vi "arm_delta.vi"(8 "Compliance [V]":dbl=0.5 format="%#_6f", 9 "DELAY [sec]":dbl=0.002 format="%#_6e", 10 "I-HIGH [A]":dbl=0.0001 format="%#_6e", 11 "Keithley":refnum<visa-resource-name>="GPIB1::20::INSTR") -> (3 "number":i32)   [LabVIEW 2019]
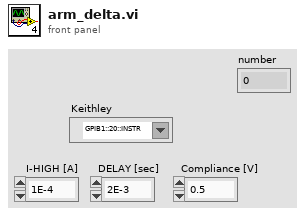
[diagram p1: front panel]
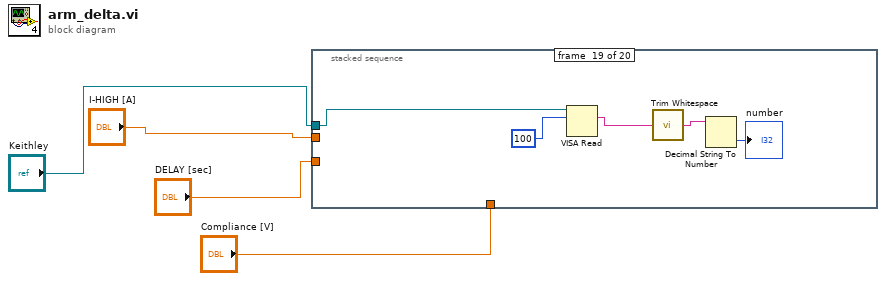
[diagram p0: block diagram]
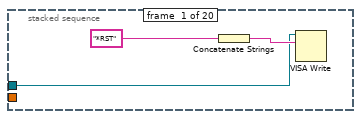
[diagram p2: hidden frame]
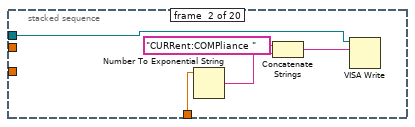
[diagram p3: hidden frame]
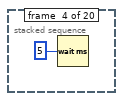
[diagram p5: hidden frame]
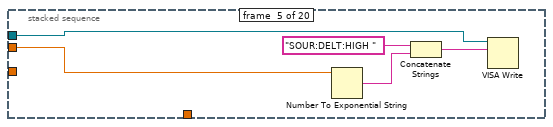
[diagram p6: hidden frame]
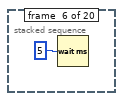
[diagram p7: hidden frame]
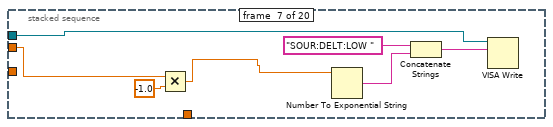
[diagram p8: hidden frame]
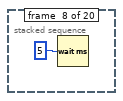
[diagram p9: hidden frame]
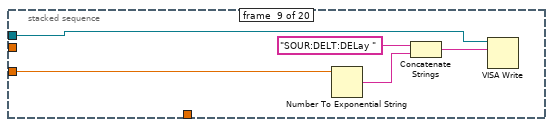
[diagram p10: hidden frame]
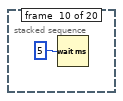
[diagram p11: hidden frame]
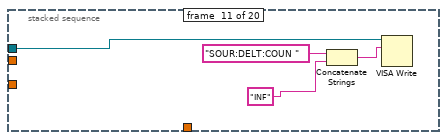
[diagram p12: hidden frame]
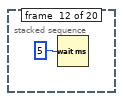
[diagram p13: hidden frame]
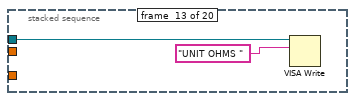
[diagram p14: hidden frame]
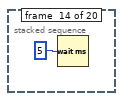
[diagram p15: hidden frame]
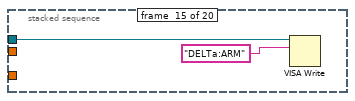
[diagram p16: hidden frame]
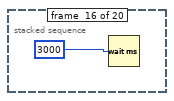
[diagram p17: hidden frame]
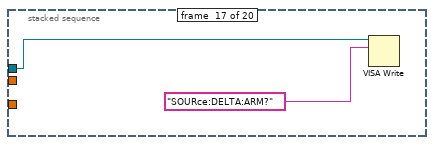
[diagram p18: hidden frame]
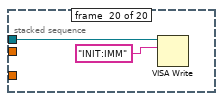
[diagram p20: hidden frame]
diagram:
  n1 = stacked-sequence {
    tunnel: "I-HIGH [A]" -> [_ _ _ _ w16 _ w20 _ _ _ _ _ _ _ _ _ _ _ _ _]
    tunnel: "Keithley" -> [w5 w9 _ _ w14 _ w23 _ w29 _ w34 _ w39 _ w42 _ w46 _ w51 w52]
    tunnel: "DELAY [sec]" -> [_ _ _ _ _ _ _ _ w28 _ _ _ _ _ _ _ _ _ _ _]
    tunnel: "Compliance [V]" -> [_ w8 _ _ _ _ _ _ _ _ _ _ _ _ _ _ _ _ _ _]
    frame #0 {
      n2 = Concatenate Strings("*RST") -> (w6:string)
      n3 = VISA Write(VISA resource name=w5, write buffer=w6) -> ()  [unwired: 1 in, 3 out]
    }
    frame #1 {
      n4 = Number To Exponential String(number=w8) -> (E-format string=w11:string)  [unwired: 3 in]
      n5 = Concatenate Strings("CURRent:COMPliance ", w11) -> (w10:string)
      n6 = VISA Write(VISA resource name=w9, write buffer=w10) -> ()  [unwired: 1 in, 3 out]
    }
    frame #2 {
    }
    frame #3 {
      n7 = Wait (ms)(milliseconds to wait=5) -> ()  [unwired: 1 out]
    }
    frame #4 {
      n8 = Number To Exponential String(number=w16) -> (E-format string=w17:string)  [unwired: 3 in]
      n9 = Concatenate Strings("SOUR:DELT:HIGH ", w17) -> (w15:string)
      n10 = VISA Write(VISA resource name=w14, write buffer=w15) -> ()  [unwired: 1 in, 3 out]
    }
    frame #5 {
      n11 = Wait (ms)(milliseconds to wait=5) -> ()  [unwired: 1 out]
    }
    frame #6 {
      n12 = Multiply(x=w20, y=-1.0) -> (x*y=w21:dbl)
      n13 = Number To Exponential String(number=w21) -> (E-format string=w25:string)  [unwired: 3 in]
      n14 = Concatenate Strings("SOUR:DELT:LOW ", w25) -> (w24:string)
      n15 = VISA Write(VISA resource name=w23, write buffer=w24) -> ()  [unwired: 1 in, 3 out]
    }
    frame #7 {
      n16 = Wait (ms)(milliseconds to wait=5) -> ()  [unwired: 1 out]
    }
    frame #8 {
      n17 = Number To Exponential String(number=w28) -> (E-format string=w31:string)  [unwired: 3 in]
      n18 = Concatenate Strings("SOUR:DELT:DELay ", w31) -> (w30:string)
      n19 = VISA Write(VISA resource name=w29, write buffer=w30) -> ()  [unwired: 1 in, 3 out]
    }
    frame #9 {
      n20 = Wait (ms)(milliseconds to wait=5) -> ()  [unwired: 1 out]
    }
    frame #10 {
      n21 = Concatenate Strings("SOUR:DELT:COUN ", "INF") -> (w36:string)
      n22 = VISA Write(VISA resource name=w34, write buffer=w36) -> ()  [unwired: 1 in, 3 out]
    }
    frame #11 {
      n23 = Wait (ms)(milliseconds to wait=5) -> ()  [unwired: 1 out]
    }
    frame #12 {
      n24 = VISA Write(VISA resource name=w39, write buffer="UNIT OHMS ") -> ()  [unwired: 1 in, 3 out]
    }
    frame #13 {
      n25 = Wait (ms)(milliseconds to wait=5) -> ()  [unwired: 1 out]
    }
    frame #14 {
      n26 = VISA Write(VISA resource name=w42, write buffer="DELTa:ARM") -> ()  [unwired: 1 in, 3 out]
    }
    frame #15 {
      n27 = Wait (ms)(milliseconds to wait=3000) -> ()  [unwired: 1 out]
    }
    frame #16 {
      n28 = VISA Write(VISA resource name=w46, write buffer="SOURce:DELTA:ARM?") -> ()  [unwired: 1 in, 3 out]
    }
    frame #17 {
    }
    frame #18 {
      n29 = VISA Read(VISA resource name=w51, byte count=100) -> (read buffer=w49:string)  [unwired: 1 in, 3 out]
      n30 = call <vilib>:"Trim Whitespace.vi"("string"=w49) -> ("trimmed string"=w48:string)  [unwired: 1 in]
      n31 = Decimal String To Number(string=w48) -> (number=→"number":i32)  [unwired: 2 in, 1 out]
    }
    frame #19 {
      n32 = VISA Write(VISA resource name=w52, write buffer="INIT:IMM") -> ()  [unwired: 1 in, 3 out]
    }
  }
